vi "Resize Image (SubVI).vi"(10 "Image Size in":T1={"Rows (X)"=256, "Colums (Y)"=256}, 11 "Refnum in":T2) -> (2 "Image Size out":T1={"Rows (X)"=256, "Colums (Y)"=256}, 3 "Refnum out":T2)   [LabVIEW 2017, in "SoC IP Library.lvlib"]
uses:
  SoC IP Library.lvlib
  <vilib>/vision/Image Controls.llb/IMAQ Image.ctl
  Controls/Image Size.ctl
  <vilib>/vision/NI_Vision_Development_Module.lvlib
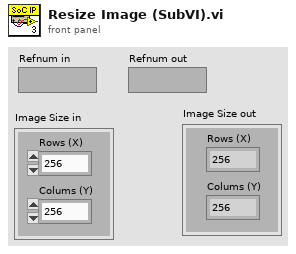
[diagram p1: front panel]
types:
  T1 = typedef "SoC IP Library.lvlib/Image Size.ctl" = cluster{"Rows (X)":u16, "Colums (Y)":u16}
  T2 = typedef "IMAQ Image.ctl" = refnum<image>
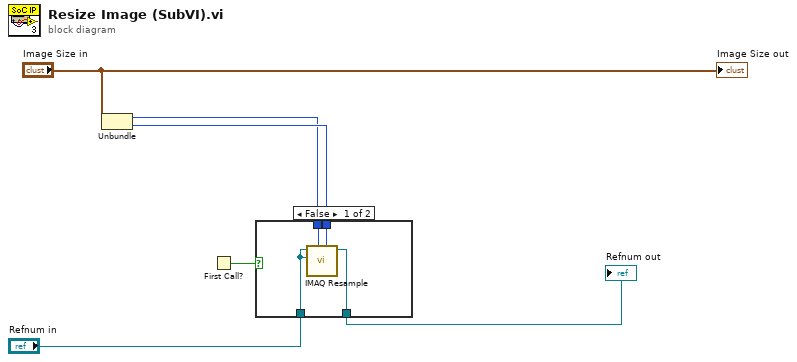
[diagram p0: block diagram]
diagram:
  n1 = Unbundle("Image Size in") -> ("Rows (X)"=w2:u16, "Colums (Y)"=w3:u16)
  n2 = First Call?() -> (First Call?: T/F=w5:bool)
  n3 = case shown="False" w5 {
    tunnel: w3 -> [w10 _]
    tunnel: "Refnum in" -> [w9 w11]
    tunnel: [w8 w11] -> w6
    tunnel: w2 -> [w7 _]
    frame False {
      n4 = call "IMAQ Resample"("X Resolution"=w10, "Y Resolution"=w7, "Image Dst"=w9, "Image Src"=w9) -> ("Image Dst Out"=w8:T2)  [unwired: 6 in, 1 out]
    }
    frame True {
    }
  }
  "Refnum out" <- w6
  "Image Size out" <- "Image Size in"
